vi "VI, Get Panel Control References.vi"(6 "error in":errorcluster, 9 "VI ref":refnum<vi>) -> (0 "error out":errorcluster, 2 "Ctl refnum array":refnum<vi>[](array[refnum]), 3 "VI ref dup":refnum<vi>)   [LabVIEW 2010]
doc: "This function gets an array of references to all the controls and indicators on a front panel."
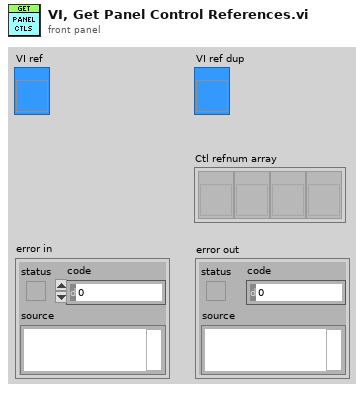
[diagram p1: front panel]
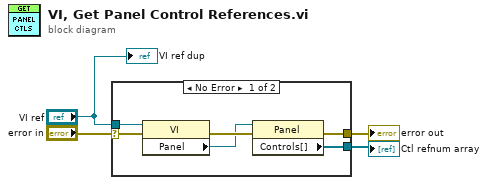
[diagram p0: block diagram]
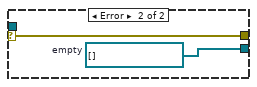
[diagram p2: hidden frame]
diagram:
  n1 = case shown="No Error" "error in" {
    selector: "error in" -> [w7 w12]
    tunnel: "VI ref" -> [w8 _]
    tunnel: [w5 w12] -> w2
    tunnel: [w6 w11] -> w1
    frame No Error {
      n2 = property class="VI"(reference=w8, error in=w7) -> (error out=w10:errorcluster, "Panel"=w9:refnum<vi>)  [unwired: 1 out]
      n3 = property class="Panel"(reference=w9, error in=w10) -> (error out=w5:errorcluster, "Controls[]"=w6:refnum<vi>[])  [unwired: 1 out]
    }
    frame Error {
      w11 = refnum<vi>[] []  # empty
    }
  }
  "error out" <- w2
  "Ctl refnum array" <- w1
  "VI ref dup" <- "VI ref"
